vi "data format_ligne 4.vi"(6 "T":waveform(dbl), 7 "Q":waveform(dbl), 8 "P":waveform(dbl)) -> (2 "spreadsheet string":string)   [LabVIEW 2014, in "PLS Logging.lvlib"]
uses:
  PLS Logging.lvlib
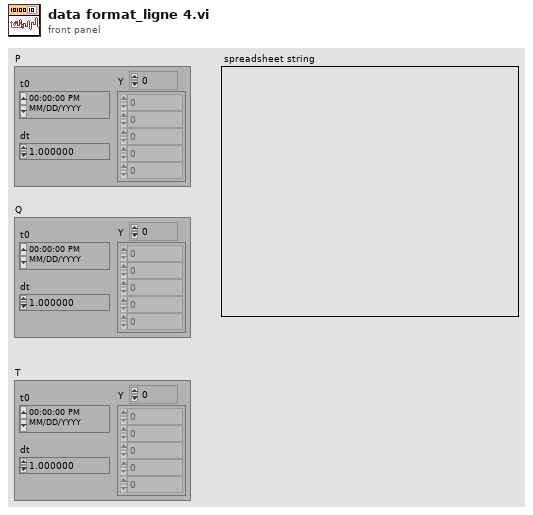
[diagram p1: front panel]
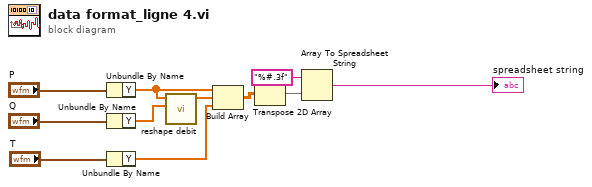
[diagram p0: block diagram]
diagram:
  n1 = Unbundle By Name("P") -> ("Y"=w10:dbl[])
  n2 = Unbundle By Name("Q") -> ("Y"=w9:dbl[])
  n3 = Unbundle By Name("T") -> ("Y"=w2:dbl[])
  n4 = call "reshape debit.vi"("Q"=w9, "P"=w10) -> ("Array"=w11:dbl[])  [unwired: 9 in]
  n5 = Build Array(w10, w11, w2) -> (w5:dbl[][])
  n6 = Transpose 2D Array(2D array=w5) -> (transposed array=w8:dbl[][])
  n7 = Array To Spreadsheet String(array=w8, 3:"%#.3f" ("format string")) -> (spreadsheet string=→"spreadsheet string":string)  [unwired: 1 in]
